vi "Real Matrix Trace.vi"(0 "Input Matrix":T1) -> (1 "trace":dbl format="%.2f", 2 "error":i32)   [LabVIEW 2017, in "NI_AALPro.lvlib"]
doc: "Finds the <B>trace</B> of <B>Input Matrix</B>. Wire data to the <B>Input Matrix</B> input to determine the polymorphic instance to use or manually select the instance."
uses:
  NI_AALPro.lvlib
  RealMatrix.ctl
  lvanlys.dll
  NI_Matrix.lvlib
panel:
  # "Trace"
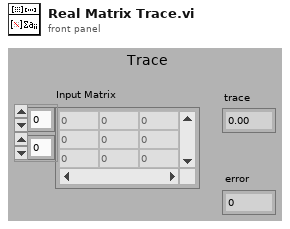
[diagram p1: front panel]
types:
  T1 = typedef "NI_Matrix.lvlib/RealMatrix.ctl" = dbl[][]
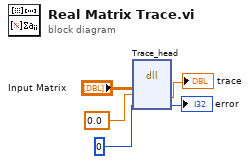
[diagram p0: block diagram]
diagram:
  n1 = dll-call lib="C:/Program Files/National Instruments/LabVIEW 2017/resource/lvanlys.*" fn="Trace_head"("Input Matrix"="Input Matrix", 0.0, 0) -> (→"trace":dbl, →"error":i32)  [unwired: 5 in, 2 out]
